vi "sub_padIQWF.vi"(1 "input complex waveform":cluster{"t0":dbl, "dt":dbl, "Y":cdb[]}, 2 "Packet Pad \n[samples]":i32) -> (0 "output complex waveform":cluster{"t0":dbl, "dt":dbl, "Y":cdb[]})   [LabVIEW 2011]
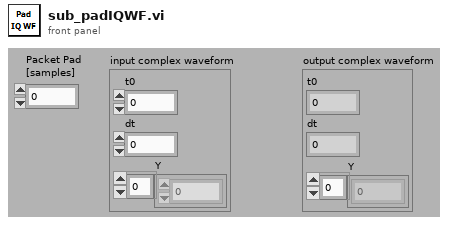
[diagram p1: front panel]
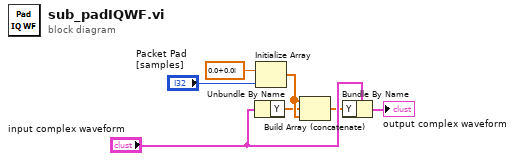
[diagram p0: block diagram]
diagram:
  n1 = Unbundle By Name("input complex waveform") -> ("Y"=w1:cdb[])
  n2 = Initialize Array(cdb 0.0+0.0i ("element"), "Packet Pad \n[samples]") -> (w4:cdb[])
  n3 = Build Array (concatenate)(w4, w1, w4) -> (w2:cdb[])
  n4 = Bundle By Name(cluster="input complex waveform", "Y"=w2) -> (→"output complex waveform":cluster{"t0":dbl, "dt":dbl, "Y":cdb[]})
